vi "RG Fetch Waveform (Waveform Data Type) with delay.vi"(8 "error in (no error)":errorcluster, 9 "Maximum Time (10000ms)":u32=10000, 10 "Channel (0: Channel 1)":u16(ring) items=["Channel 1", "Channel 2", "Channel 3", "Channel 4", "Math", "Reference 1", "Reference 2", "Reference 3", "Reference 4", "D0", "D1", "D2", "D3", "D4", "D5", "D6", "D7", "D8", "D9", "D10", "D11", "D12", "D13", "D14", "D15", "Amplitude", "Frequency", "Phase", "Normal", "Average", "Maximum Peak Hold", "Minimum Peak Hold"], 11 "VISA resource name":refnum<visa-resource-name>) -> (0 "error out":errorcluster, 2 "Waveform Data":waveform(dbl)(graph), 3 "VISA resource name out":refnum<visa-resource-name>)   [LabVIEW 2017, in "Scope.lvlib" / "Tektronix DPO MSO 2000 4000 Series.lvlib"]
doc: "Returns the waveform that an oscilloscope acquires for a channel you specify. An acquisition that you initiate before calling this VI generates the waveform.\n\nYou first enable channels with the Configure Channel VI. Then you use the Initiate VI to start an acquisition on the enabled channels. An oscilloscope concurrently acquires waveforms for these channels. You must call the Fetch Waveform VI separately to obtain waveforms for each enabled channel.\nHowever, you also can call the Read Waveform VI instead of using the above low-level VIs.\n\n<B>Note</B>: Use the Fetch Waveform VI only with other low-level VIs, such as the Initiate VI, the Abort VI, and the Fetch Waveform Measurement VI. High-level VIs, such as the Read Waveform VI, automatically incorporate the functions of the Initiate VI and the Fetch Waveform VI. The Fetch Waveform VI does not check the status of an instrument."
uses:
  Tektronix DPO MSO 2000 4000 Series.lvlib
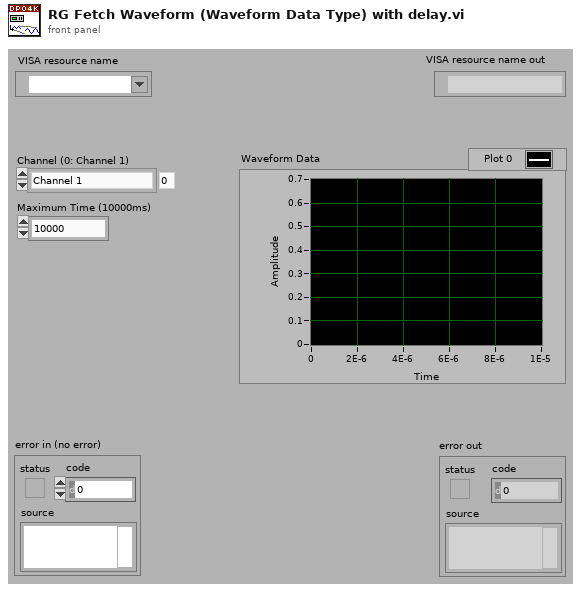
[diagram p1: front panel]
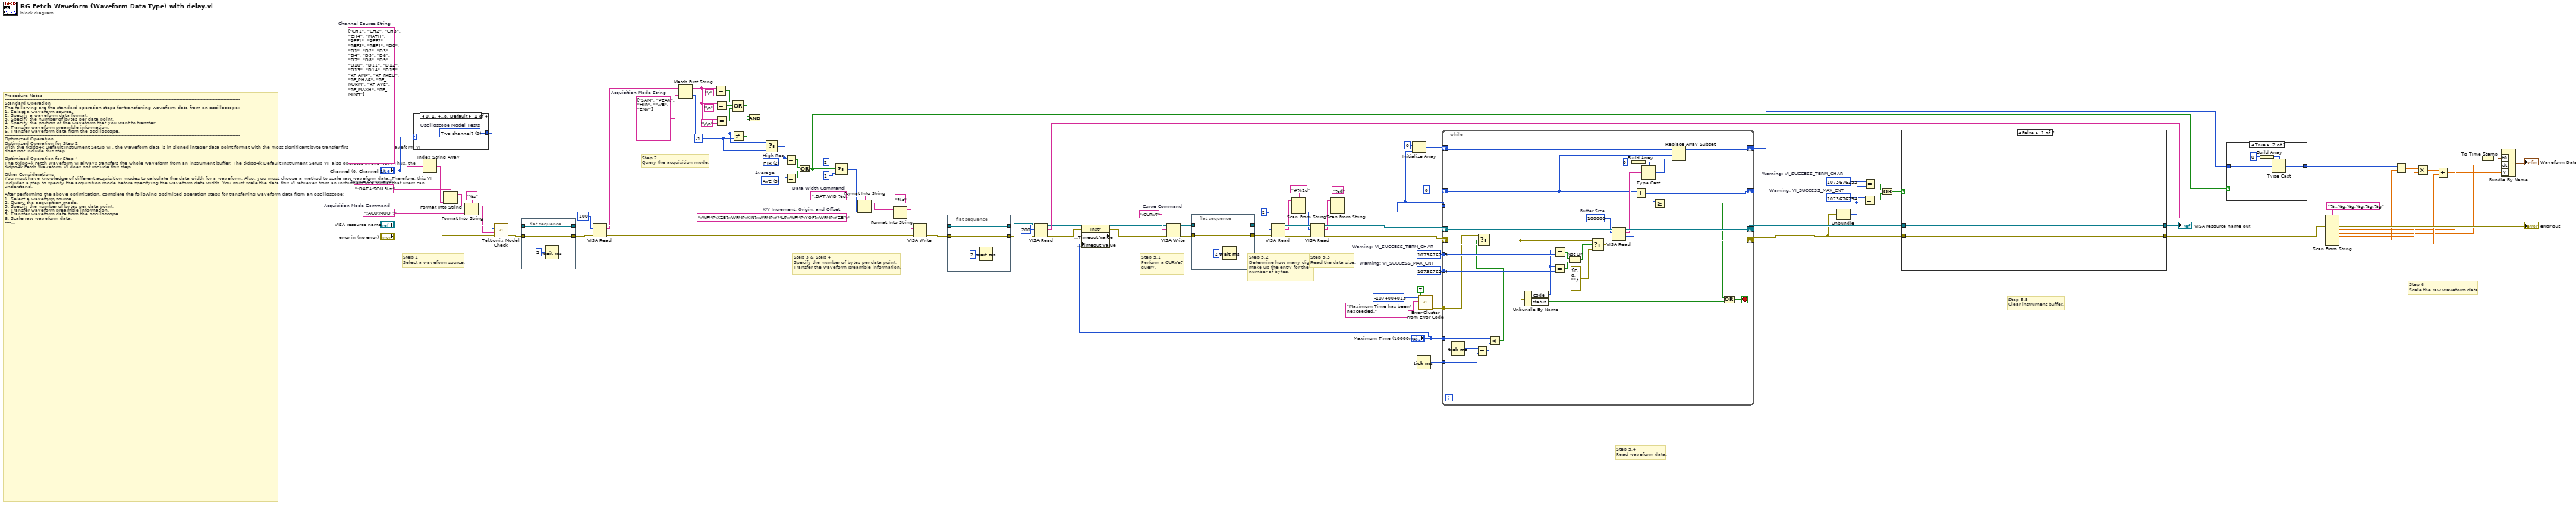
[diagram p0: block diagram]
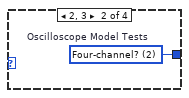
[diagram p2: hidden frame]
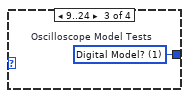
[diagram p3: hidden frame]
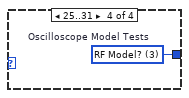
[diagram p4: hidden frame]
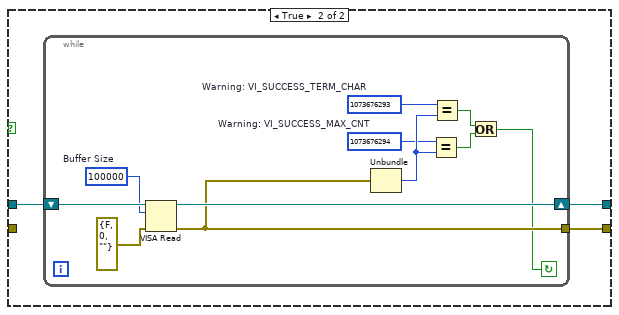
[diagram p6: hidden frame]
diagram:
  w49 = 1073676294  # Warning: VI_SUCCESS_MAX_CNT
  w50 = 1073676293  # Warning: VI_SUCCESS_TERM_CHAR
  w53 = 1073676294  # Warning: VI_SUCCESS_MAX_CNT
  w52 = 1073676293  # Warning: VI_SUCCESS_TERM_CHAR
  w62 = -1 ("y")
  w88 = ":CURV?"  # Curve Command
  w96 = ":DAT:WID %d;"  # Data Width Command
  w101 = u16 3 items=["SAM", "PEAK", "HIR", "AVE", "ENV"]  # Average
  w102 = u16 2 items=["SAM", "PEAK", "HIR", "AVE", "ENV"]  # High Res
  w74 = string[] ["SAM", "PEAK", "HIR", "AVE", "ENV"]  # Acquisition Mode String
  w95 = ":ACQ:MOD?;"  # Acquisition Mode Command
  w107 = string[] ["CH1", "CH2", "CH3", "CH4", "MATH", "REF1", "REF2", "REF3", "REF4", "D0", "D1", "D2", "D3", "D4", "D5", "D6", "D7", "D8", "D9", "D10", "D11", "D12", "D13", "D14", "D15", "RF_AMP", "RF_FREQ", "RF_PHAS", "RF_NORM", "RF_AVE", "RF_MAXH", "RF_MINH"]  # Channel Source String
  w106 = ":DATA:SOU %s;"  # Source Command
  w93 = ":WFMP:XZE?;:WFMP:XIN?;:WFMP:YMU?;:WFMP:YOF?;:WFMP:YZE?;"  # X/Y Increment, Origin, and Offset
  # "Step 6    \nScale the raw waveform data."
  # "Step 5.5    \nClear instrument buffer."
  # "Step 5.4   \nRead waveform data."
  # "Step 5.3      \nRead the data size."
  # "Step 5.2      \nDetermine how many digits\nmake up the entry for the \nnumber of bytes."
  # "Step 5.1      \nPerform a CURVe?\nquery."
  # "Step 3 & Step 4         \nSpecify the number of bytes per data point.\nTransfer the waveform preamble information."
  # "Step 2        \nQuery the acquisition mode."
  # "Step 1 \nSelect a waveform source."
  # "Procedure Notes\n-----------------------------------------------------------------------------------------------------------------------------------------------------------\nStandard Operation\nThe following are the standard operation steps for transferring waveform data from an oscilloscope:\n1. Select a waveform source.\n2. Specify a waveform data format.\n3. Specify the number of bytes per data point.\n4. Specify the portion of the waveform that you want to transfer.\n5. Transfer waveform preamble information.\n6. Transfer waveform data from the oscilloscope.\n-----------------------------------------------------------------------------------------------------------------------------------------------------------\nOptimized Operation\nOptimized Operation for Step 2\nWith the tkdpo4k Default Instrument Setup VI , the waveform data is in signed integer data point format with the most significant byte transfer first. Thus, the Fetch Waveform VI does not include this step . \n\nOptimized Operation for Step 4 \nThe tkdpo4k Fetch Waveform VI always transfers the whole waveform from an instrument buffer. The tkdpo4k Default Instrument Setup VI  also operates in this way. Thus, the tkdpo4k Fetch Waveform VI does not include this step. \n\nOther Considerations\nYou must have knowledge of different acquisition modes to calculate the data width for a waveform. Also, you must choose a method to scale raw waveform data. Therefore, this VI includes a step to specify the acquisition mode before specifying the waveform data width. You must scale the data this VI retrieves from an instrument to a format that users can understand.\n\nAfter performing the above optimization, complete the following optimized operation steps for transferring waveform data from an oscilloscope:\n1. Select a waveform source.\n2. Query the acquisition mode.\n3. Specify the number of bytes per data point.\n4. Transfer waveform preamble information.\n5. Transfer waveform data from the oscilloscope.\n6. Scale raw waveform data.\n-----------------------------------------------------------------------------------------------------------------------------------------------------------\nDetailed Steps\nThe following steps detail the behavior of this VI:\n1. Select a waveform source. \n2. Query and determine the acquisition mode. A correct determination is critical to steps 3 and 6.\n    -----------------------------------------------\n    Acquisition Mode |  Data Width   \n    -----------------------------------------------\n    Normal                       |   1                      \n    -----------------------------------------------\n    Peak Detect               |   1                      \n    -----------------------------------------------\n    Hi Res                        |   2                      \n    -----------------------------------------------\n    Envelope                   |   1                      \n    ----------------------------------------------- \n    Average                    |   2                      \n    -----------------------------------------------\n3. Specify the number of bytes per data point. For the Hi Res or Average acquisition modes, set the data width to 2. For all other acquisition modes, set the data width to 1.\n4. Transfer the waveform preamble information. Necessary preamble information includes XZero, XIncrement, YMultiplier, YOffset, and YZero. This VI uses XZero and XIncrement to configure the x-axis of output waveforms and uses YMultiplier, YOffset, and YZero to scale data values. This VI then parses the return string of the preamble query in step 6.\n5. Transfer waveform data from the oscilloscope.\n    5.1 Perform a CURVe? query.\n    5.2 Determine how many digits make up the entry for the number of bytes.\n    5.3 Read the data size.\n    5.4 Call the VISA Read VI repeatedly with a buffer size of 10000 until you obtain as much data as the data size specifies. Use      an 8-bit array to store the raw waveform data you obtain. \n    5.5 Continue reading the data remaining in the instrument buffer until the buffer is empty.\n6. Scale the raw waveform data.\n    6.1 Cast the waveform data to a 16-bit array if the data width is 2 . Split the waveform data into a minimum and a maximum data array if the acquisition mode is Peak Detect or Envelope. This VI skips this step if the data width is 1.\n    6.2 Parse the preamble information.\n    6.3 Scale the waveform data according to the following formula:\n          Data_Value_in_units = (Raw_Data_Value - YOffset) * YMultiplier + YZero\n          The resulting waveform data has a unit of volts.\n    6.4 Build a waveform graph."
  n1 = case shown="0, 1, 4..8, Default" "Channel (0: Channel 1)" {
    tunnel: [w108 w109 w110 w111] -> w17
    frame 0, 1, 4..8, Default {
      w108 = u16 0 items=["Two-channel?", "Digital Model?", "Four-channel?", "RF Model?"]  # Oscilloscope Model Tests
    }
    frame 2, 3 {
      w109 = u16 2 items=["Two-channel?", "Digital Model?", "Four-channel?", "RF Model?"]  # Oscilloscope Model Tests
    }
    frame 9..24 {
      w110 = u16 1 items=["Two-channel?", "Digital Model?", "Four-channel?", "RF Model?"]  # Oscilloscope Model Tests
    }
    frame 25..31 {
      w111 = u16 3 items=["Two-channel?", "Digital Model?", "Four-channel?", "RF Model?"]  # Oscilloscope Model Tests
    }
  }
  n2 = Index String Array(1:"Channel (0: Channel 1)", 2:w107) -> (0:w105:string)  [unwired: 1 in]
  n3 = Format Into String(format string=w106, w105) -> (resulting string=w104:string)  [unwired: 2 in, 1 out]
  n4 = Format Into String(format string="%s", initial string=w104, w95) -> (resulting string=w20:string)  [unwired: 1 in, 1 out]
  n5 = call "Tektronix Model Check.vi"("error in (no error)"="error in (no error)", "Command String"=w20, "Oscilloscope Model Tests (3: RF Model?)"=w17, "VISA resource name"="VISA resource name") -> ("error out"=w14:errorcluster, "VISA resource name out"=w16:refnum<visa-resource-name>)  [unwired: 6 in]
  n6 = flat-sequence {
    tunnel: w16 -> [w114]
    tunnel: [w114] -> w15
    tunnel: w14 -> [w113]
    tunnel: [w113] -> w13
    frame #0 {
      n7 = Wait (ms)(milliseconds to wait=u32 2) -> ()  [unwired: 1 out]
    }
  }
  n8 = VISA Read(VISA resource name=w15, byte count=u32 100, error in (no error)=w13) -> (VISA resource name out=w92:refnum<visa-resource-name>, read buffer=w73:string, error out=w91:errorcluster)  [unwired: 1 out]
  n9 = Match First String(2:w74, 3:w73) -> (0:w63:i32, 1:w69:string)
  n10 = Equal?(x=w69, y="\r") -> (x = y?=w68:bool)
  n11 = Equal?(x=w69, y="\n") -> (x = y?=w67:bool)
  n12 = Equal?(x=w69, y="\r\n") -> (x = y?=w66:bool)
  n13 = Not Equal?(x=w63, y=w62) -> (x != y?=w64:bool)
  n14 = Compound Arithmetic op=OR(w68, w67, w66) -> (w65:bool)
  n15 = And(x=w65, y=w64) -> (x .and. y?=w61:bool)
  n16 = Select(t=w63, s=w61, f=w62) -> (s? t:f=w48:i32)
  n17 = Equal?(x=w48, y=w102) -> (x = y?=w100:bool)
  n18 = Equal?(x=w48, y=w101) -> (x = y?=w99:bool)
  n19 = Or(x=w100, y=w99) -> (x .or. y?=w47:bool)
  n20 = Select(t=2 ("f"), s=w47, f=1) -> (s? t:f=w79:i32)
  n21 = Format Into String(format string=w96, w79) -> (resulting string=w90:string)  [unwired: 2 in, 1 out]
  n22 = Format Into String(format string="%s", initial string=w90, w93) -> (resulting string=w80:string)  [unwired: 1 in, 1 out]
  n23 = VISA Write(VISA resource name=w92, write buffer=w80, error in (no error)=w91) -> (VISA resource name out=w12:refnum<visa-resource-name>, error out=w10:errorcluster)  [unwired: 1 out]
  n24 = flat-sequence {
    tunnel: w12 -> [w116]
    tunnel: [w116] -> w11
    tunnel: w10 -> [w115]
    tunnel: [w115] -> w9
    frame #0 {
      n25 = Wait (ms)(milliseconds to wait=u32 2) -> ()  [unwired: 1 out]
    }
  }
  n26 = VISA Read(VISA resource name=w11, byte count=u32 200, error in (no error)=w9) -> (VISA resource name out=w28:refnum<visa-resource-name>, read buffer=w78:string, error out=w27:errorcluster)  [unwired: 1 out]
  n27 = property class="Instr" props=["General Settings:Timeout Value", "General Settings:Timeout Value"](reference=w28, error in=w27, "General Settings:Timeout Value"="Maximum Time (10000ms)") -> (reference out=w26:refnum<visa-resource-name>, error out=w25:errorcluster)  [unwired: 1 out]
  n28 = VISA Write(VISA resource name=w26, write buffer=w88, error in (no error)=w25) -> (VISA resource name out=w8:refnum<visa-resource-name>, error out=w7:errorcluster)  [unwired: 1 out]
  n29 = flat-sequence {
    tunnel: w8 -> [w119]
    tunnel: [w119] -> w5
    tunnel: w7 -> [w118]
    tunnel: [w118] -> w6
    frame #0 {
      n30 = Wait (ms)(milliseconds to wait=u32 2) -> ()  [unwired: 1 out]
    }
  }
  n31 = VISA Read(VISA resource name=w5, byte count=u32 2, error in (no error)=w6) -> (VISA resource name out=w85:refnum<visa-resource-name>, read buffer=w83:string, error out=w84:errorcluster)  [unwired: 1 out]
  n32 = Scan From String(format string="#%1d", input string=w83) -> (output 1=w82:i32)  [unwired: 3 in, 3 out]
  n33 = VISA Read(VISA resource name=w85, byte count=w82, error in (no error)=w84) -> (VISA resource name out=w24:refnum<visa-resource-name>, read buffer=w4:string, error out=w23:errorcluster)  [unwired: 1 out]
  n34 = Scan From String(format string="%d", input string=w4) -> (output 1=w60:i32)  [unwired: 3 in, 3 out]
  n35 = Initialize Array(i8 0 ("element"), w60) -> (w58:i8[])
  n36 = Tick Count (ms)() -> (millisecond timer value=w33:u32)
  n37 = call <vilib>:"Error Cluster From Error Code.vi"("show call chain? (False)"=TRUE, "error message (\"\")"="Maximum Time has been\nexceeded." ("error message (\"\")"), "error code (0)"=-1074004013) -> ("error out"=w29:errorcluster)  [unwired: 6 in]
  n38 = while {
    shift-right: [w151] -> w2
    shift-left: w24 -> [w153]
    shift-right: [w150] -> w1
    shift-left: w23 -> [w123]
    shift-right: [w146] -> w46
    shift-left: w58 -> [w147]
    tunnel: w60 -> [w143]
    shift-right: [w140] -> _
    shift-left: 0 -> [w141]
    tunnel: w50 -> [w134]
    tunnel: w49 -> [w133]
    tunnel: w33 -> [w127]
    tunnel: "Maximum Time (10000ms)" -> [w125]
    tunnel: w29 -> [w122]
    stop <- w139 stop-if-true
    w152 = 100000  # Buffer Size
    n39 = Tick Count (ms)() -> (millisecond timer value=w128:u32)
    n40 = Subtract(x=w128, y=w127) -> (x-y=w126:u32)
    n41 = Less?(x=w125, y=w126) -> (x < y?=w121:bool)
    n42 = Select(t=w122, s=w121, f=w123) -> (s? t:f=w124:errorcluster)
    n43 = Unbundle By Name(w124) -> ("code"=w132:i32, "status"=w136:bool)
    n44 = Equal?(x=w132, y=w133) -> (x = y?=w130:bool)
    n45 = Equal?(x=w132, y=w134) -> (x = y?=w131:bool)
    n46 = Not Or(1:w130, 2:w131) -> (0:w129:bool)
    n47 = Select(t=w124, s=w129, f=errorcluster {"status"=FALSE, "code"=0, "source"=""} ("error in (no error)")) -> (s? t:f=w135:errorcluster)
    n48 = VISA Read(VISA resource name=w153, byte count=w152, error in (no error)=w135) -> (VISA resource name out=w151:refnum<visa-resource-name>, read buffer=w145:string, return count=w144:u32, error out=w150:errorcluster)
    n49 = Build Array(i8 0) -> (w149:i8[])
    n50 = Add(x=w141, y=w144) -> (x+y=w140:u32)
    n51 = Type Cast(type=w149, x=w145) -> (*(type *) &x=w142:i8[])
    n52 = Greater Or Equal?(x=w140, y=w143) -> (x >= y?=w138:bool)
    n53 = Replace Array Subset(array=w147, new element=w142, index=w141) -> (w146:i8[])
    n54 = Compound Arithmetic op=OR(w138, w136) -> (w139:bool)
  }
  n55 = Unbundle(w1) -> ("code"=w54:i32)  [unwired: 2 out]
  n56 = Equal?(x=w53, y=w54) -> (x = y?=w56:bool)
  n57 = Equal?(x=w52, y=w54) -> (x = y?=w57:bool)
  n58 = Or(x=w57, y=w56) -> (x .or. y?=w55:bool)
  n59 = case shown="False" w55 {
    tunnel: w2 -> [w155 w158]
    tunnel: w1 -> [w154 _]
    tunnel: [w155 w157] -> w75
    tunnel: [w154 w156] -> w77
    frame False {
    }
    frame True {
      n60 = while {
        shift-right: [w168] -> w157
        shift-left: w158 -> [w169]
        tunnel: [w161] -> w156
        stop <- w160 continue-if-true
        w163 = 1073676294  # Warning: VI_SUCCESS_MAX_CNT
        w162 = 1073676293  # Warning: VI_SUCCESS_TERM_CHAR
        w167 = u32 100000  # Buffer Size
        n61 = VISA Read(VISA resource name=w169, byte count=w167, error in (no error)=errorcluster {"status"=FALSE, "code"=0, "source"=""}) -> (VISA resource name out=w168:refnum<visa-resource-name>, error out=w161:errorcluster)  [unwired: 2 out]
        n62 = Unbundle(w161) -> ("code"=w164:i32)  [unwired: 2 out]
        n63 = Equal?(x=w163, y=w164) -> (x = y?=w165:bool)
        n64 = Equal?(x=w162, y=w164) -> (x = y?=w166:bool)
        n65 = Or(x=w166, y=w165) -> (x .or. y?=w160:bool)
      }
    }
  }
  "VISA resource name out" <- w75
  n66 = case shown="True" w47 {
    tunnel: w46 -> [w170 w172]
    tunnel: [w170 w171] -> w35
    frame False {
    }
    frame True {
      n67 = Build Array(i16 0 ("element")) -> (w173:i16[])
      n68 = Type Cast(type=w173, x=w172) -> (*(type *) &x=w171:i16[])
    }
  }
  n69 = Scan From String(format string="%.;%g;%g;%g;%g;%g", input string=w78, error in=w77) -> (error out=→"error out":errorcluster, output 1=w39:dbl, output 2=w38:dbl, output 3=w40:dbl, output 4=w41:dbl, output 5=w42:dbl)  [unwired: 6 in, 2 out]
  n70 = Subtract(x=w35, y=w41) -> (x-y=w44:dbl[])
  n71 = Multiply(x=w44, y=w40) -> (x*y=w43:dbl[])
  n72 = Add(x=w43, y=w42) -> (x+y=w37:dbl[])
  n73 = To Time Stamp(1:w39) -> (0:w36:timestamp)
  n74 = Bundle By Name("t0"=w36, "dt"=w38, "Y"=w37) -> (→"Waveform Data":waveform(dbl))  [unwired: 1 in]
